vi "路径查找创建-报警记录清单-网络版.vi"() -> (0 "累积剂量数据库":path, 1 "蜂鸣音效文件路径":path, 3 "Client 版帮助文档路径":path, 4 "探头属性配置文件":path, 5 "配置文件":path, 6 "缓存数据文件夹":path, 7 "远程控制exe":path, 8 "导出记录":path, 9 "短信通知配置文件":path, 10 "报警记录清单":path, 11 "Server 版帮助文档路径":path, 12 "状态栏信息文件":path, 14 "报表模板":path, 15 "报表文件夹":path)   [LabVIEW 2017]
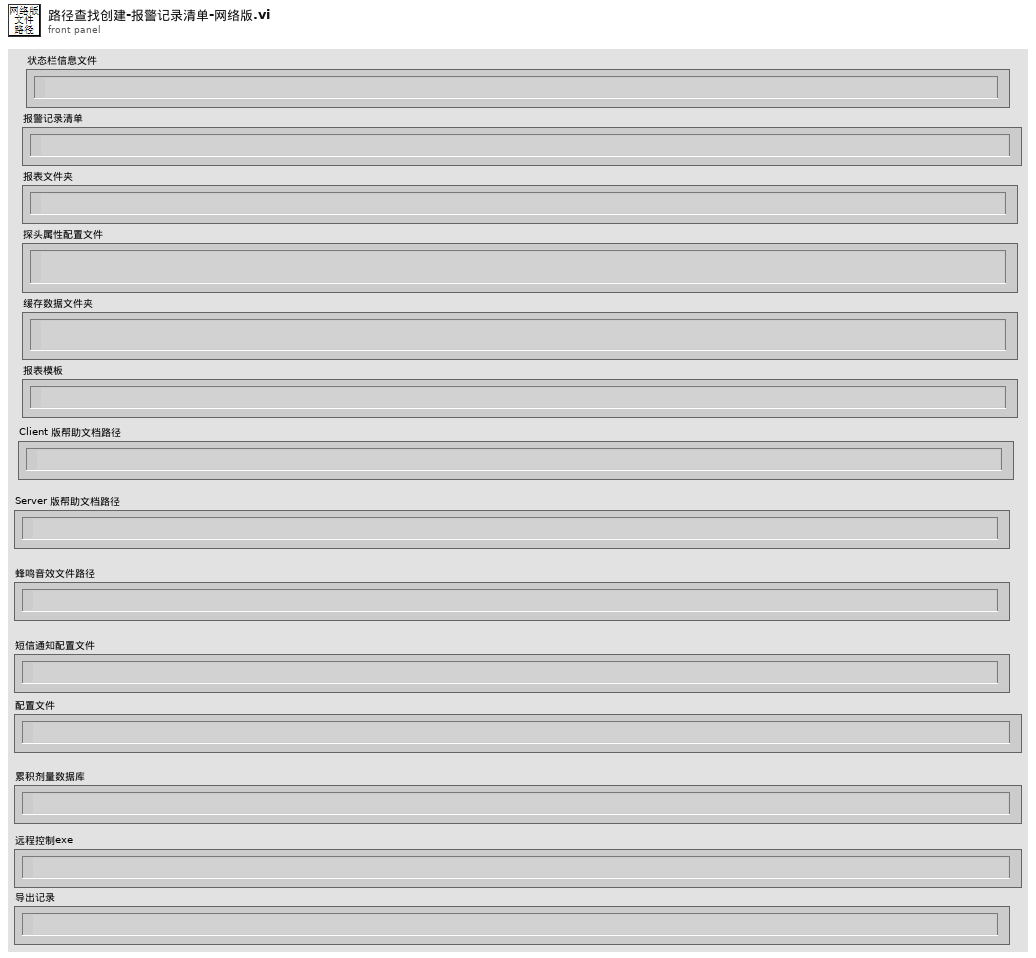
[diagram p1: front panel]
types:
  T1 = enum16{"open", "replace", "create", "open or create", "replace or create", "replace or create with confirmation"}
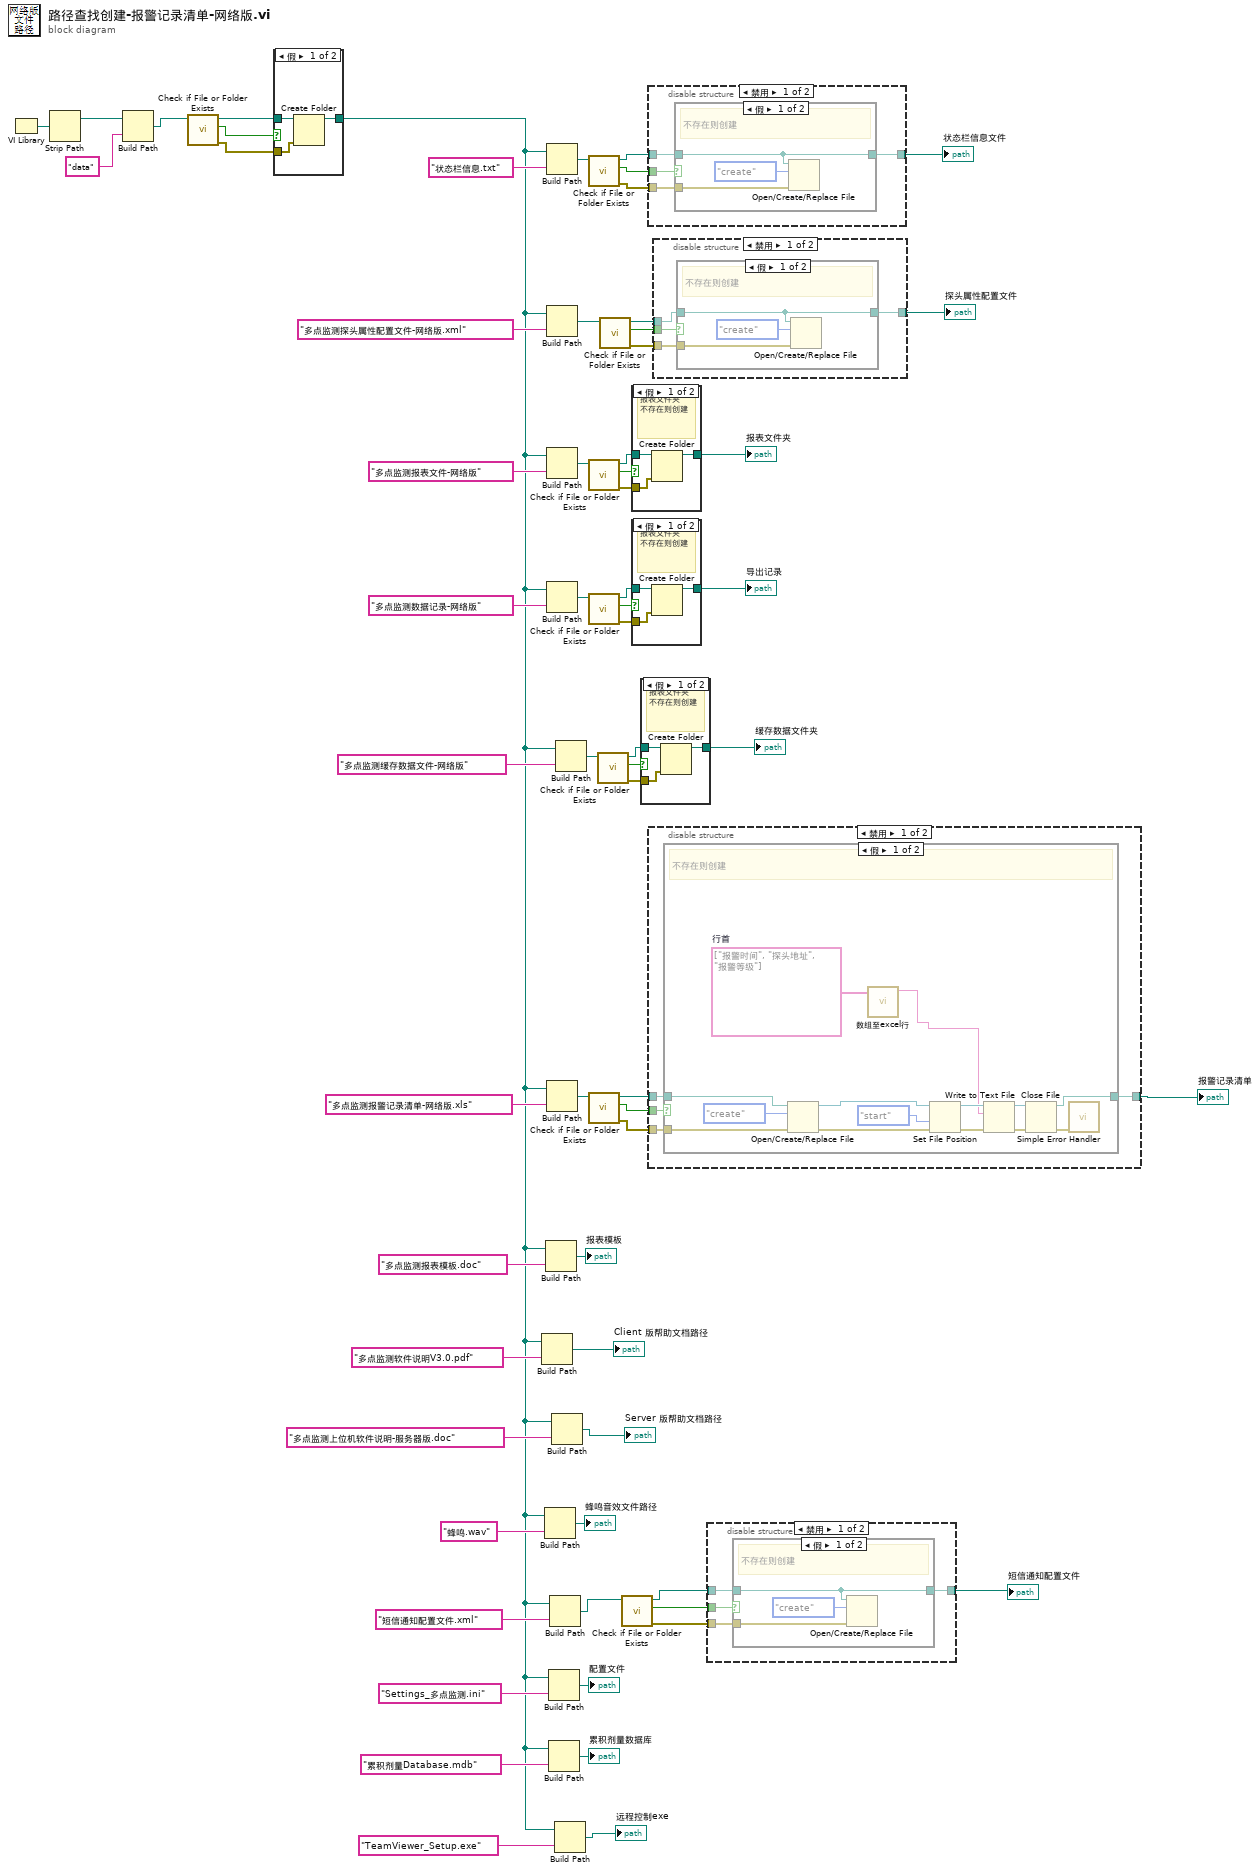
[diagram p0: block diagram]
diagram:
  n1 = VI Library() -> (path=w60:path)
  n2 = Strip Path(path=w60) -> (stripped path=w14:path)  [unwired: 1 out]
  n3 = Build Path(base path=w14, name or relative path="data" ("读报警文件")) -> (appended path=w10:path)
  n4 = call <vilib>:"Check if File or Folder Exists.vi"("path"=w10) -> ("error out"=w11:errorcluster, "file or folder exists?"=w12:bool, "dup path"=w13:path)  [unwired: 8 in]
  n5 = case shown="假" w12 {
    tunnel: w13 -> [w67 w68]
    tunnel: w11 -> [w66 _]
    tunnel: [w65 w68] -> w2
    frame False {
      n6 = Create Folder(path (use dialog)=w67, error in=w66) -> (created path=w65:path)  [unwired: 1 in, 2 out]
    }
    frame True {
    }
  }
  n7 = Build Path(base path=w2, name or relative path="多点监测软件说明V3.0.pdf" ("读报警文件")) -> (appended path=→"Client 版帮助文档路径":path)
  n8 = Build Path(base path=w2, name or relative path="蜂鸣.wav" ("读报警文件")) -> (appended path=→"蜂鸣音效文件路径":path)
  n9 = Build Path(base path=w2, name or relative path="多点监测报表模板.doc" ("读报警文件")) -> (appended path=→"报表模板":path)
  n10 = Build Path(base path=w2, name or relative path="状态栏信息.txt" ("读报警文件")) -> (appended path=w35:path)
  n11 = Build Path(base path=w2, name or relative path="多点监测探头属性配置文件-网络版.xml" ("读报警文件")) -> (appended path=w47:path)
  n12 = Build Path(base path=w2, name or relative path="多点监测报表文件-网络版" ("读报警文件")) -> (appended path=w56:path)
  n13 = Build Path(base path=w2, name or relative path="多点监测数据记录-网络版" ("读报警文件")) -> (appended path=w4:path)
  n14 = Build Path(base path=w2, name or relative path="多点监测报警记录清单-网络版.xls" ("读报警文件")) -> (appended path=w63:path)
  n15 = Build Path(base path=w2, name or relative path="Settings_多点监测.ini" ("读报警文件")) -> (appended path=→"配置文件":path)
  n16 = Build Path(base path=w2, name or relative path="累积剂量Database.mdb" ("读报警文件")) -> (appended path=→"累积剂量数据库":path)
  n17 = Build Path(base path=w2, name or relative path="短信通知配置文件.xml" ("读报警文件")) -> (appended path=w21:path)
  n18 = Build Path(base path=w2, name or relative path="多点监测上位机软件说明-服务器版.doc" ("读报警文件")) -> (appended path=→"Server 版帮助文档路径":path)
  n19 = Build Path(base path=w2, name or relative path="TeamViewer_Setup.exe" ("名称或相对路径")) -> (appended path=→"远程控制exe":path)
  n20 = Build Path(base path=w2, name or relative path="多点监测缓存数据文件-网络版" ("读报警文件")) -> (appended path=w41:path)
  n21 = call <vilib>:"Check if File or Folder Exists.vi"("path"=w35) -> ("error out"=w33:errorcluster, "file or folder exists?"=w31:bool, "dup path"=w32:path)  [unwired: 8 in]
  n22 = call <vilib>:"Check if File or Folder Exists.vi"("path"=w56) -> ("error out"=w53:errorcluster, "file or folder exists?"=w55:bool, "dup path"=w54:path)  [unwired: 8 in]
  n23 = call <vilib>:"Check if File or Folder Exists.vi"("path"=w4) -> ("error out"=w7:errorcluster, "file or folder exists?"=w5:bool, "dup path"=w6:path)  [unwired: 8 in]
  n24 = call <vilib>:"Check if File or Folder Exists.vi"("path"=w63) -> ("error out"=w62:errorcluster, "file or folder exists?"=w59:bool, "dup path"=w61:path)  [unwired: 8 in]
  n25 = call <vilib>:"Check if File or Folder Exists.vi"("path"=w41) -> ("error out"=w44:errorcluster, "file or folder exists?"=w42:bool, "dup path"=w43:path)  [unwired: 8 in]
  n26 = call <vilib>:"Check if File or Folder Exists.vi"("path"=w47) -> ("error out"=w48:errorcluster, "file or folder exists?"=w50:bool, "dup path"=w49:path)  [unwired: 8 in]
  n27 = call <vilib>:"Check if File or Folder Exists.vi"("path"=w21) -> ("error out"=w24:errorcluster, "file or folder exists?"=w22:bool, "dup path"=w23:path)  [unwired: 8 in]
  n28 = case shown="假" w55 {
    tunnel: w54 -> [w71 w72]
    tunnel: w53 -> [w70 _]
    tunnel: [w69 w72] -> w52
    frame False {
      # "报表文件夹\n不存在则创建"
      n29 = Create Folder(path (use dialog)=w71, error in=w70) -> (created path=w69:path)  [unwired: 1 in, 2 out]
    }
    frame True {
    }
  }
  "报表文件夹" <- w52
  n30 = case shown="假" w5 {
    tunnel: w6 -> [w75 w76]
    tunnel: w7 -> [w74 _]
    tunnel: [w73 w76] -> w1
    frame False {
      # "报表文件夹\n不存在则创建"
      n31 = Create Folder(path (use dialog)=w75, error in=w74) -> (created path=w73:path)  [unwired: 1 in, 2 out]
    }
    frame True {
    }
  }
  "导出记录" <- w1
  n32 = case shown="假" w42 {
    tunnel: w43 -> [w79 w80]
    tunnel: w44 -> [w78 _]
    tunnel: [w77 w80] -> w45
    frame False {
      # "报表文件夹\n不存在则创建"
      n33 = Create Folder(path (use dialog)=w79, error in=w78) -> (created path=w77:path)  [unwired: 1 in, 2 out]
    }
    frame True {
    }
  }
  "缓存数据文件夹" <- w45
  n34 = disable-structure shown="禁用" {
    disable-tunnel: w33 -> [w84 _]
    disable-tunnel: w32 -> [w83 _]
    disable-tunnel: w31 -> [w82 _]
    disable-tunnel: [w81 _] -> w30
    frame Disabled {
      n35 = case shown="假" w82 {
        tunnel: w84 -> [w86 _]
        tunnel: w83 -> [w85 w88]
        tunnel: [w85 w88] -> w81
        frame False {
          # "不存在则创建"
          n36 = Open/Create/Replace File(file path (use dialog)=w85, error in=w86, operation (0:open)=T1."create" ("操作(0:open)")) -> ()  [unwired: 3 in, 3 out]
        }
        frame True {
          # "存在则输出"
        }
      }
    }
    frame Enabled {
    }
  }
  "状态栏信息文件" <- w30
  n37 = disable-structure shown="禁用" {
    disable-tunnel: w62 -> [w92 _]
    disable-tunnel: w61 -> [w91 _]
    disable-tunnel: w59 -> [w90 _]
    disable-tunnel: [w89 _] -> w58
    frame Disabled {
      n38 = case shown="假" w90 {
        tunnel: w92 -> [w105 _]
        tunnel: w91 -> [w104 w107]
        tunnel: [w95 w107] -> w89
        frame False {
          w94 = string[] ["报警时间", "探头地址", "报警等级"]  # 行首
          # "不存在则创建"
          n39 = Open/Create/Replace File(file path (use dialog)=w104, error in=w105, operation (0:open)=T1."create" ("操作(0:open)")) -> (refnum out=w97:refnum<file>, error out=w96:errorcluster)  [unwired: 3 in, 1 out]
          n40 = call "数组至excel行.vi"("数组"=w94) -> ("字符串"=w93:string)  [unwired: 10 in]
          n41 = Set File Position(refnum=w97, from (0:start)=enum16{"start", "end", "current"}."start" ("自（0:起始）"), error in=w96) -> (refnum out=w100:refnum<file>, error out=w99:errorcluster)  [unwired: 1 out]
          n42 = Write to Text File(file (use dialog)=w100, text=w93, error in=w99) -> (refnum out=w102:refnum<file>, error out=w103:errorcluster)  [unwired: 2 out]
          n43 = Close File(refnum=w102, error in=w103) -> (path=w95:path, error out=w101:errorcluster)
          n44 = call <vilib>:"Simple Error Handler.vi"("error in (no error)"=w101) -> ()  [unwired: 1 in, 8 out]
        }
        frame True {
          # "存在则输出"
        }
      }
    }
    frame Enabled {
    }
  }
  "报警记录清单" <- w58
  n45 = disable-structure shown="禁用" {
    disable-tunnel: [w111 _] -> w51
    disable-tunnel: w50 -> [w110 _]
    disable-tunnel: w49 -> [w109 _]
    disable-tunnel: w48 -> [w108 _]
    frame Disabled {
      n46 = case shown="假" w110 {
        tunnel: w108 -> [w113 _]
        tunnel: w109 -> [w112 w115]
        tunnel: [w112 w115] -> w111
        frame False {
          # "不存在则创建"
          n47 = Open/Create/Replace File(file path (use dialog)=w112, error in=w113, operation (0:open)=T1."create" ("操作(0:open)")) -> ()  [unwired: 3 in, 3 out]
        }
        frame True {
          # "存在则输出"
        }
      }
    }
    frame Enabled {
    }
  }
  "探头属性配置文件" <- w51
  n48 = disable-structure shown="禁用" {
    disable-tunnel: w24 -> [w119 _]
    disable-tunnel: w23 -> [w118 _]
    disable-tunnel: w22 -> [w117 _]
    disable-tunnel: [w116 _] -> w20
    frame Disabled {
      n49 = case shown="假" w117 {
        tunnel: w119 -> [w121 _]
        tunnel: w118 -> [w120 w123]
        tunnel: [w120 w123] -> w116
        frame False {
          # "不存在则创建"
          n50 = Open/Create/Replace File(file path (use dialog)=w120, error in=w121, operation (0:open)=T1."create" ("操作(0:open)")) -> ()  [unwired: 3 in, 3 out]
        }
        frame True {
          # "存在则输出"
        }
      }
    }
    frame Enabled {
    }
  }
  "短信通知配置文件" <- w20
